vi "magnetoresistance with smu.vi"() -> ()   [LabVIEW 2017]
doc: "Use this template to build a simple state machine design pattern. Each state executes code and determines which state to transition to."
uses:
  magnetoresistance/controls/State.ctl
  <vilib>/DAQmx/create/channels.llb/DAQmx Create Channel (AI-Voltage-Basic).vi
  <vilib>/DAQmx/configure/trigger.llb/DAQmx Start Trigger (None).vi
  <vilib>/Utility/error.llb/DialogType.ctl
  <vilib>/DAQmx/write.llb/DAQmx Write (Analog DBL 1Chan 1Samp).vi
  magnetoresistance/controls/Instruments.ctl
  magnetoresistance/controls/State_of_loop.ctl
  magnetoresistance/controls/Data.ctl
  <vilib>/DAQmx/configure/timing.llb/DAQmx Timing (Sample Clock).vi
  <vilib>/DAQmx/create/channels.llb/DAQmx Create Channel (AO-Voltage-Basic).vi
panel:
  out "Type of magnet":bool
  in  "Number of loops":i32=1 caption="Stop H Field (Oe)" min=0
  in  "Time to wait, ms":i32=100 caption="Stop H Field (Oe)" min=0
  in  "Clear button":bool
  in  "Data Type":T1(ring)=enum."Resistance, Ohm"
  out "Ush.Min":dbl=-5.0
  out "Ush.Max":dbl=5.0
  out "U.Min":dbl=-5.0
  out "U.Max":dbl=5.0
  in  "Load resistance, Ohm":dbl=24000.0 min=0.0
  in  "Switch port":refnum<visa-resource-name>="COM6"
  in  "AKIP":refnum<visa-resource-name>="AKIP"
  in  "Resolution, Oe/point":dbl=100.0 caption="Stop H Field (Oe)" min=0.0 format="%#_6f"
  out "DC power electromagnet":cluster{"Voltage":dbl, "Current":dbl}={"Voltage"=0.00544, "Current"=0.05} {"Voltage" format="%.2f"; "Current" format="%.2f"}
  out "Error Out":errorcluster={"status"=FALSE, "code"=1073676293, "source"="VISA Read in AKIP_read.vi->AKIP_error_check.vi->AKIP_reset_errors.vi->magnetoresistance.vi"}
  in  "Error In (no error)":errorcluster
  in  "Voltage Output, V":dbl=2.5 min=0.0 max=5.0
  in  "H Field Max, Oe":dbl=2000.0 caption="Stop H Field (Oe)" min=0.0 max=6000.0 format="%#_6f"
  in  "H Field Min, Oe":dbl=-2000.0 min=-6000.0 max=0.0 format="%#_6f"
  out "Status":string="Shutting down..."
  in  "Exit Button":bool
  in  "Save Button":bool
  out "Cursor":cluster{"x":dbl, "y":dbl} {"x" format="%.2f"; "y" format="%.5f"}
  out "SpectrumGraph":cluster{"Old Field":dbl[], "Old Signal":dbl[]}[](graph)
  in  "Start Button":bool
  in  "Stop Button":bool
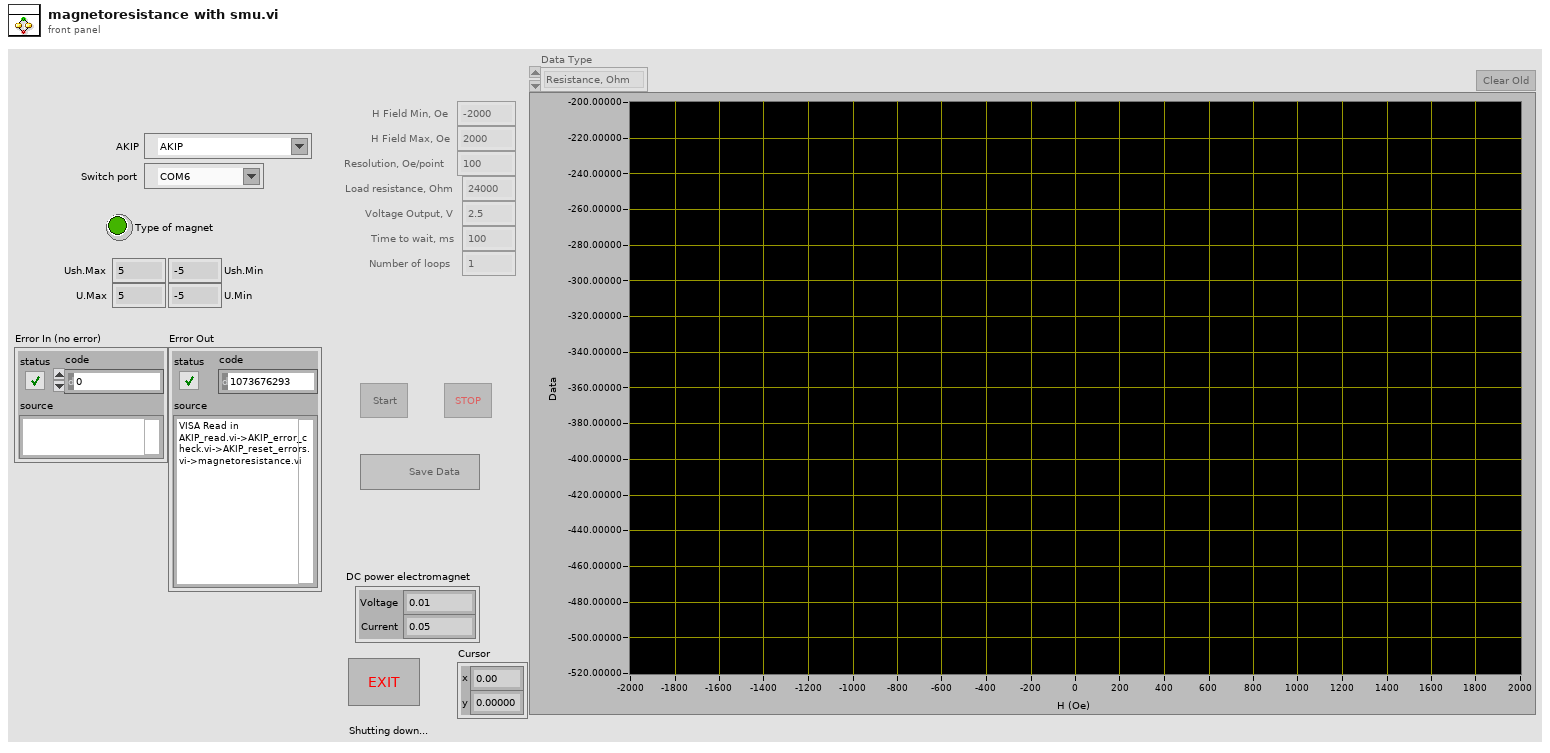
[diagram p1: front panel]
types:
  T1 = enum16{"Voltage Ush, V", "Voltage U, V", "Sum Voltage, V", "Current, mA", "Resistance, Ohm"}
  T2 = typedef "Data.ctl" = cluster{"Field":dbl[], "Voltage Ush":dbl[], "Voltage U":dbl[], "Sum Voltage":dbl[], "Current":dbl[], "Resistance":dbl[], "Old Field":dbl[], "Old Voltage Ush":dbl[], "Old Voltage U":dbl[], "Old Sum Voltage":dbl[], "Old Current":dbl[], "Old Resistance":dbl[]}
  T3 = typedef "State_of_loop.ctl" = enum16{"from zero to max", "from max to zero", "from zero to min", "from min to zero"}
  T4 = typedef "Instruments.ctl" = cluster{"DAQ AO task":refnum<k21>, "DAQ AI task":refnum<k21>, "DAQ channel Voltage Output":tag, "DAQ channel Voltage U":tag, "DAQ channel Voltage Ush":tag, "AKIP":refnum<visa-resource-name>, "Switch port":refnum<visa-resource-name>}
  T5 = typedef "State.ctl" = enum16{"Init", "Idle", "Starting meas", "Running", "Stopping meas", "Shutdown"}
  T6 = cluster{"Old Field":dbl[], "Old Resistance":dbl[]}[]
  T7 = cluster{"Voltage Ush":dbl, "Voltage U":dbl, "Sum Voltage":dbl, "Current":dbl, "Resistance":dbl}
  T8 = typedef "DialogType.ctl" = u16
  T9 = typedef "LVPoint32TypeDef.ctl" = cluster{"Horizontal":i32, "Vertical":i32}
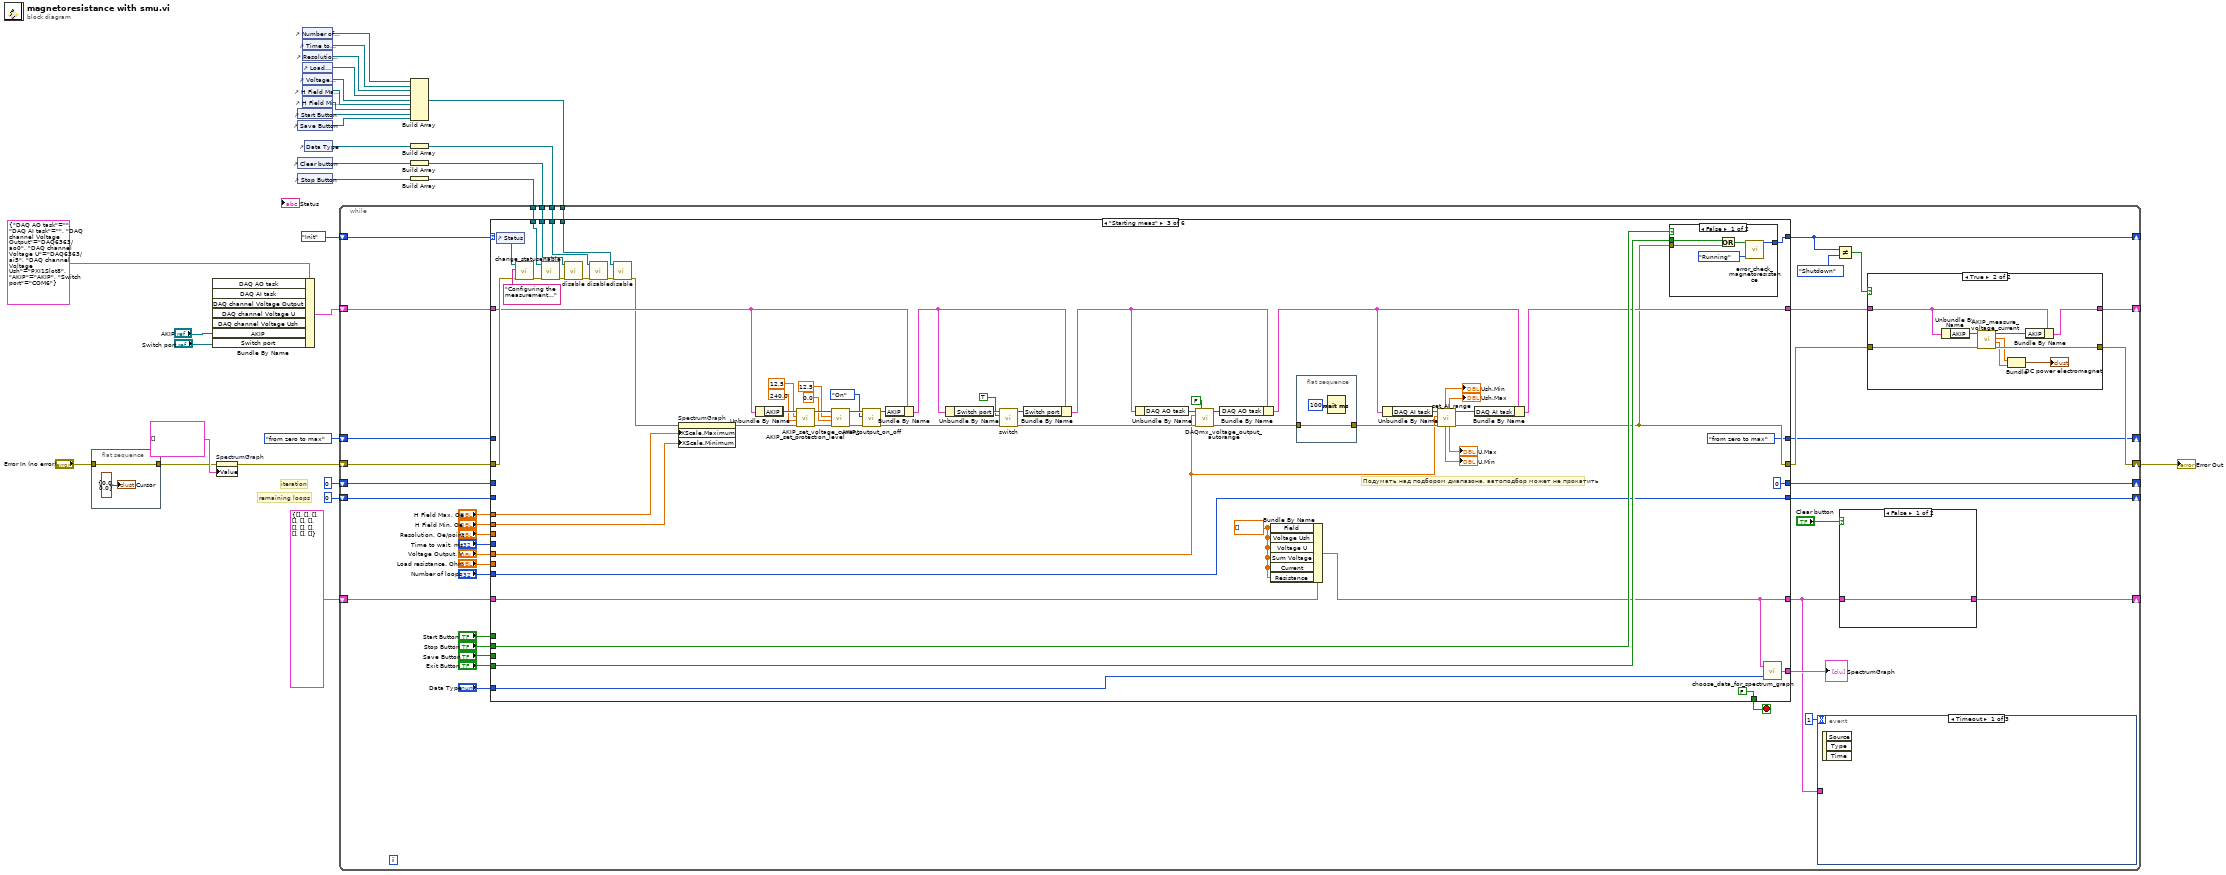
[diagram p0: block diagram]
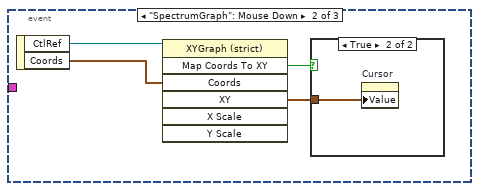
[diagram p3: hidden frame]
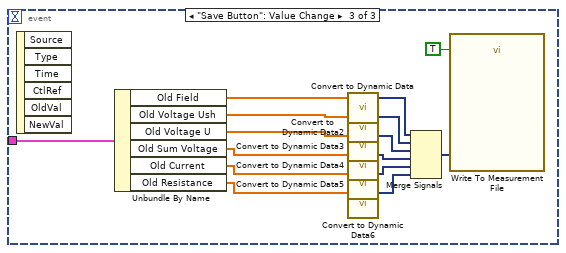
[diagram p5: hidden frame]
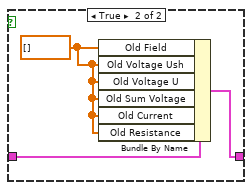
[diagram p6: hidden frame]
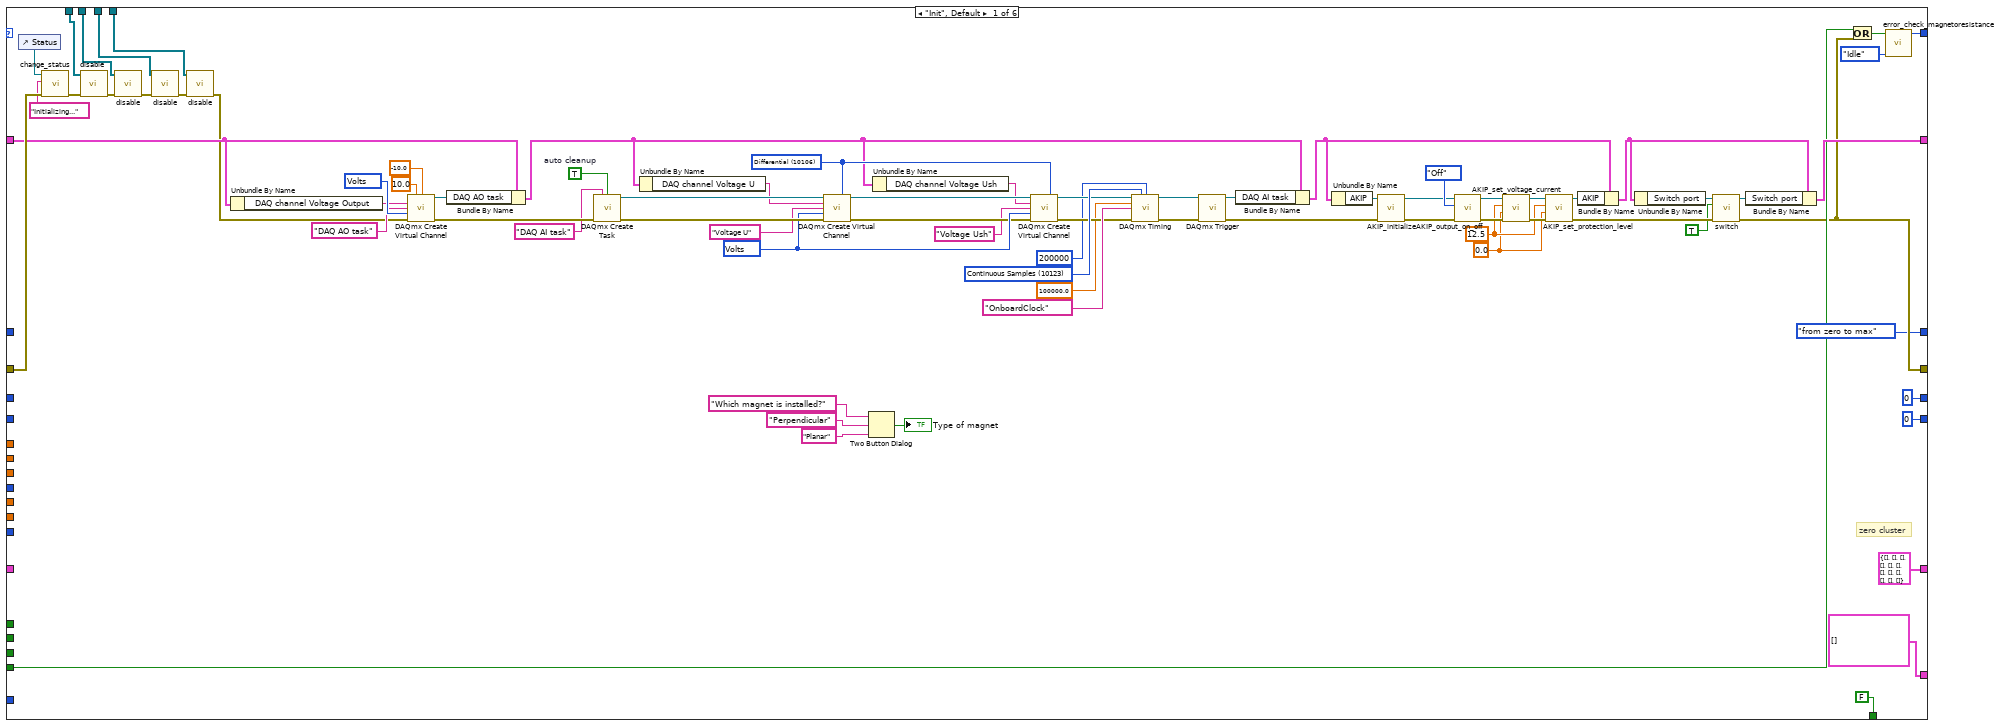
[diagram p7: hidden frame]
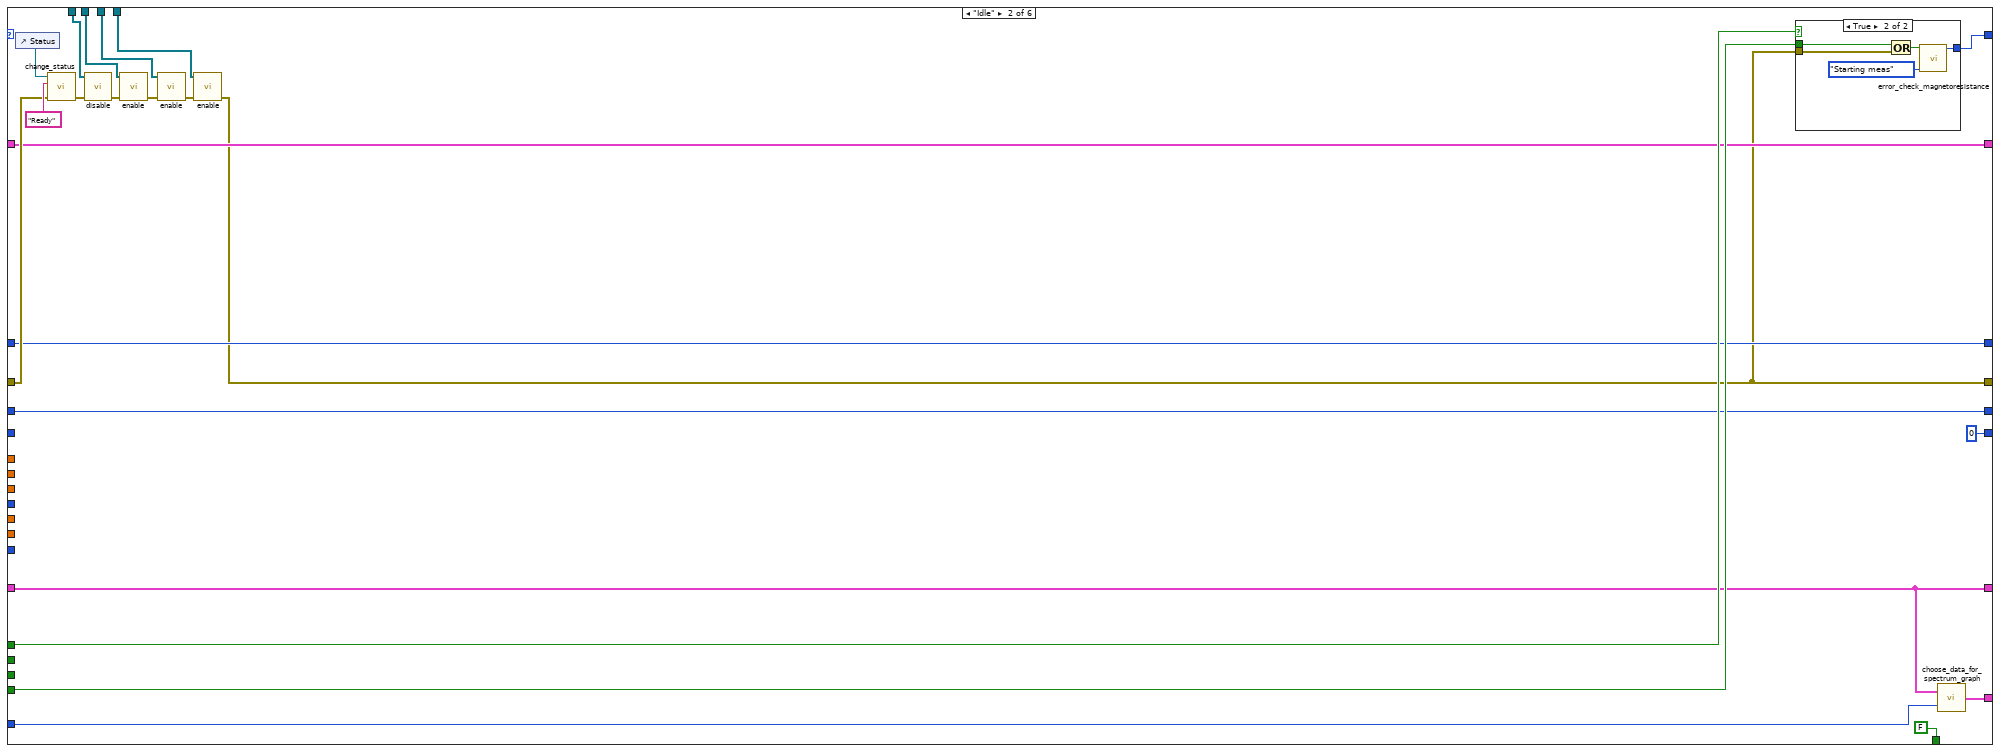
[diagram p8: hidden frame]
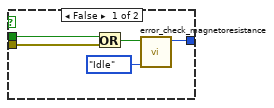
[diagram p9: hidden frame]
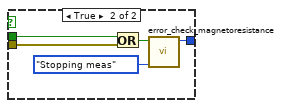
[diagram p10: hidden frame]
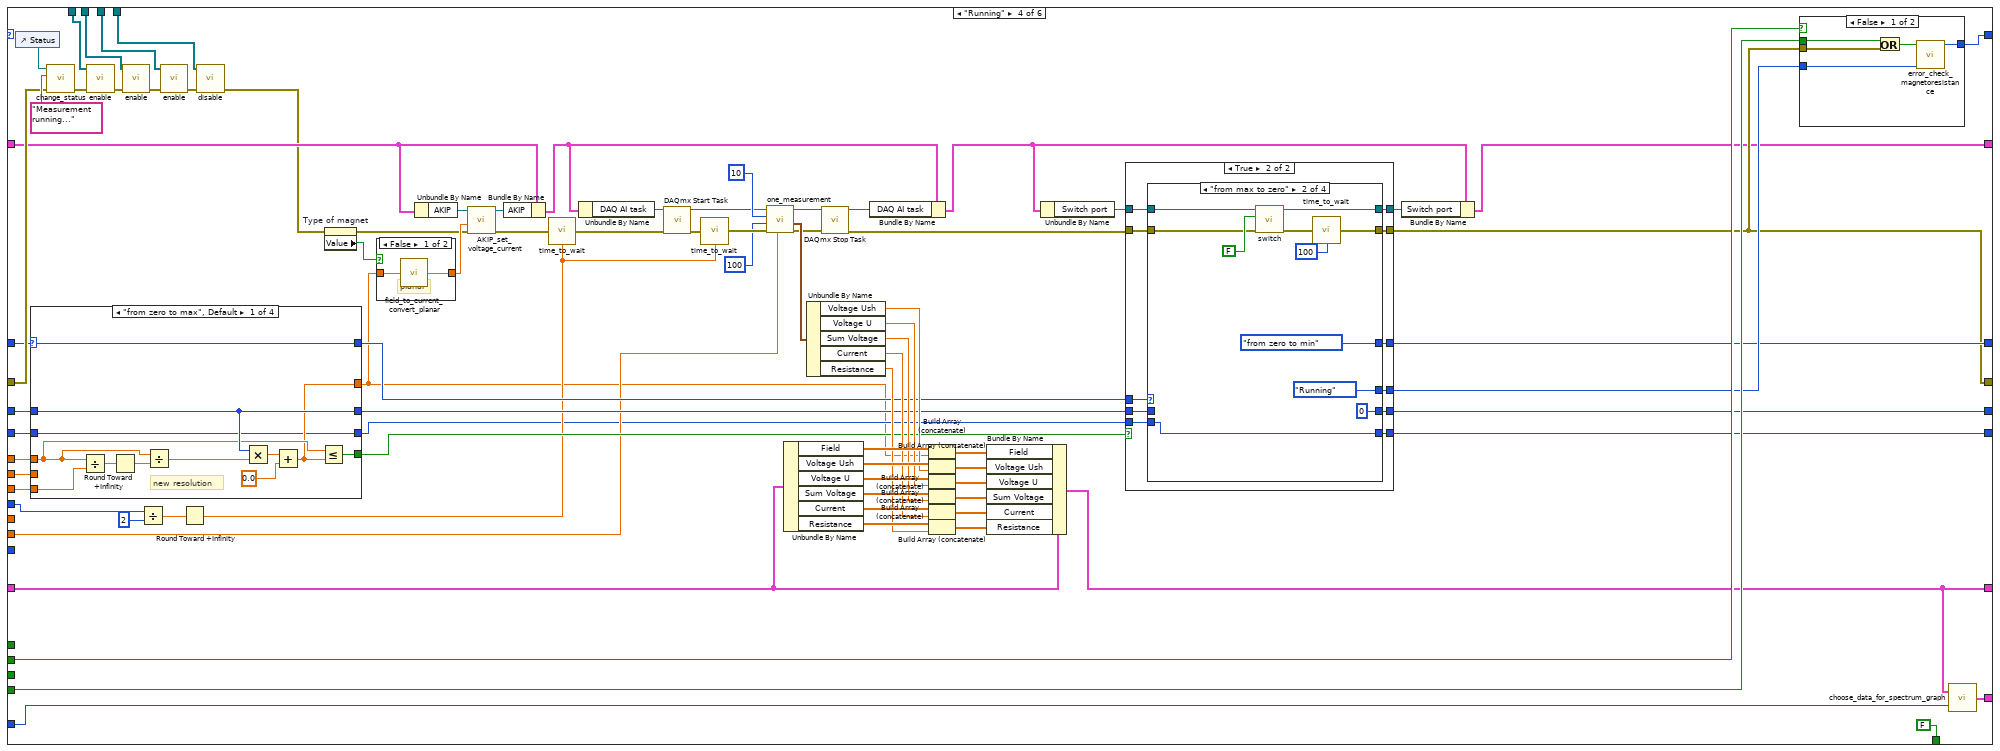
[diagram p11: hidden frame]
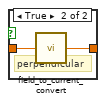
[diagram p12: hidden frame]
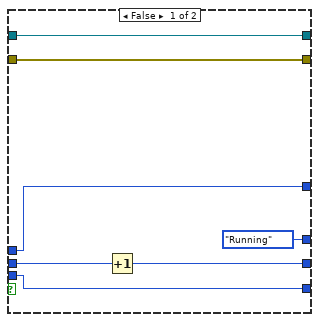
[diagram p13: hidden frame]
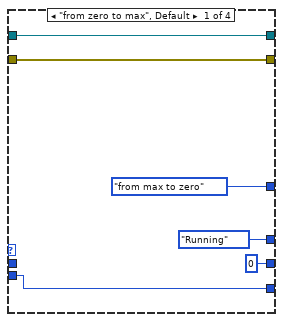
[diagram p14: hidden frame]
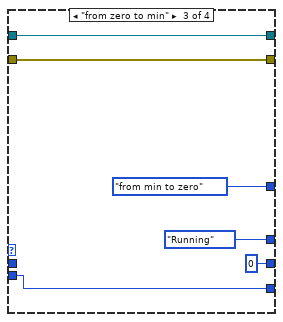
[diagram p15: hidden frame]
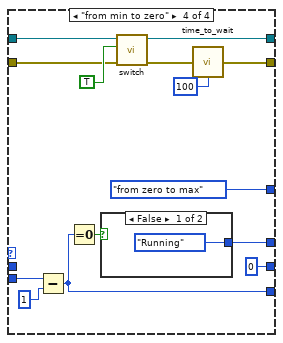
[diagram p16: hidden frame]
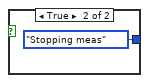
[diagram p17: hidden frame]
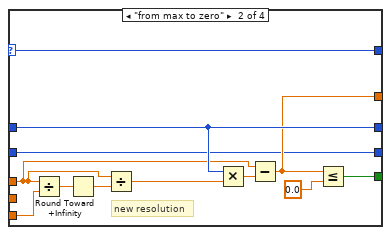
[diagram p18: hidden frame]
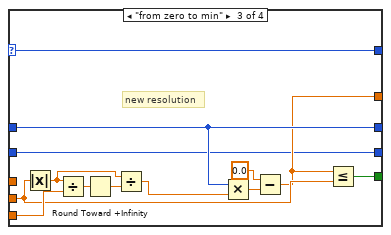
[diagram p19: hidden frame]
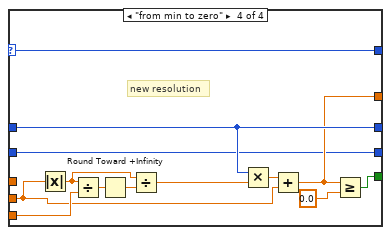
[diagram p20: hidden frame]
diagram:
  # "iteration"
  # "remaining loops"
  n1 = flat-sequence {
    tunnel: "Error In (no error)" -> [w32]
    tunnel: [w32] -> w19
    frame #0 {
      "Cursor" <- cluster{"x":dbl, "y":dbl} {"x"=0.0, "y"=0.0} ("Cursor")
    }
  }
  n2 = Bundle By Name(cluster=T4 {"DAQ AO task"="", "DAQ AI task"="", "DAQ channel Voltage Output"="DAQ6363/ao0", "DAQ channel Voltage U"="DAQ6363/ai5", "DAQ channel Voltage Ush"="PXI1Slot8", "AKIP"="AKIP", "Switch port"="COM6"} ("Cluster"), "AKIP"="AKIP", "Switch port"="Switch port") -> (w16:T4)  [unwired: 5 in]
  n3 = property on="SpectrumGraph" class="XYGraph (strict)"(error in=w19, "Value"=cluster{"Old Field":dbl[], "Old Signal":dbl[]}[] [] ("SpectrumGraph")) -> (error out=w23:errorcluster)  [unwired: 1 in, 1 out]
  n4 = control-ref of="Start Button"() -> (w28:refnum<vi>)
  n5 = control-ref of="Save Button"() -> (w27:refnum<vi>)
  n6 = control-ref of="Clear button"() -> (w10:refnum<vi>)
  n7 = control-ref of="Stop Button"() -> (w26:refnum<vi>)
  n8 = control-ref of="Number of loops"() -> (w1:refnum<vi>)
  n9 = control-ref of="Time to wait, ms"() -> (w3:refnum<vi>)
  n10 = control-ref of="Resolution, Oe/point"() -> (w4:refnum<vi>)
  n11 = control-ref of="Load resistance, Ohm"() -> (w5:refnum<vi>)
  n12 = control-ref of="Voltage Output, V"() -> (w6:refnum<vi>)
  n13 = control-ref of="H Field Max, Oe"() -> (w30:refnum<vi>)
  n14 = control-ref of="H Field Min, Oe"() -> (w29:refnum<vi>)
  n15 = control-ref of="Data Type"() -> (w9:refnum<vi>)
  n16 = Build Array(w1, w3, w4, w5, w6, w30, w29, w28, w27) -> (w24:refnum<vi>[])
  n17 = Build Array(w9) -> (w8:refnum<vi>[])
  n18 = Build Array(w10) -> (w7:refnum<vi>[])
  n19 = Build Array(w26) -> (w25:refnum<vi>[])
  n20 = while {
    tunnel: w25 -> [w71]
    tunnel: w24 -> [w70]
    shift-right: [w39] -> _
    shift-left: State."Init" ("States") -> [w64]
    shift-right: [w58] -> w15
    shift-left: w23 -> [w69]
    shift-right: [w60] -> _
    shift-left: w16 -> [w62]
    shift-right: [w51] -> _
    shift-left: State_of_loop."from zero to max" -> [w52]
    shift-right: [w49] -> _
    shift-left: 0 -> [w50]
    shift-right: [w44] -> _
    shift-left: T2 {"Field"=[], "Voltage Ush"=[], "Voltage U"=[], "Sum Voltage"=[], "Current"=[], "Resistance"=[], "Old Field"=[], "Old Voltage Ush"=[], "Old Voltage U"=[], "Old Sum Voltage"=[], "Old Current"=[], "Old Resistance"=[]} ("SpectrumGraph") -> [w48]
    tunnel: w7 -> [w41]
    tunnel: w8 -> [w40]
    shift-right: [w33] -> _
    shift-left: 0 -> [w34]
    stop <- w63 stop-if-true
    n21 = case shown="\"Starting meas\"" w64 {
      tunnel: w71 -> [w117 w187 w226 w309 w502 w552]
      tunnel: w70 -> [w114 w184 w223 w306 w499 w549]
      tunnel: w69 -> [w181 w204 w275 w368 w545 w599]
      tunnel: "Start Button" -> [_ w202 _ _ _ _]
      tunnel: "Stop Button" -> [_ _ w250 w366 _ _]
      tunnel: "Save Button" -> [_ _ _ _ _ _]
      tunnel: "Exit Button" -> [w124 w201 w249 w365 w518 _]
      tunnel: [w175 w200 w251 w367 w519 State."Shutdown" ("States out")] -> w39
      tunnel: [FALSE FALSE FALSE FALSE FALSE TRUE] -> w63
      tunnel: w62 -> [w167 w198 w240 w356 w493 w582]
      tunnel: [w125 w198 w247 w321 w497 w574] -> w61
      tunnel: [w123 w188 w246 w325 w496 w581] -> w59
      tunnel: "Load resistance, Ohm" -> [_ _ _ w297 _ _]
      tunnel: "H Field Max, Oe" -> [_ _ w220 w361 _ _]
      tunnel: "H Field Min, Oe" -> [_ _ w219 w360 _ _]
      tunnel: "Voltage Output, V" -> [_ _ w217 _ _ _]
      tunnel: "Resolution, Oe/point" -> [_ _ _ w359 _ _]
      tunnel: w52 -> [_ w197 _ w364 _ _]
      tunnel: [State_of_loop."from zero to max" w197 State_of_loop."from zero to max" w326 State_of_loop."from zero to max" State_of_loop."from zero to max"] -> w51
      tunnel: w50 -> [_ w193 _ w363 _ _]
      tunnel: [0 w193 0 w330 0 0] -> w49
      tunnel: w48 -> [_ w194 w244 w338 w509 _]
      tunnel: [T2 {"Field"=[], "Voltage Ush"=[], "Voltage U"=[], "Sum Voltage"=[], "Current"=[], "Resistance"=[], "Old Field"=[], "Old Voltage Ush"=[], "Old Voltage U"=[], "Old Sum Voltage"=[], "Old Current"=[], "Old Resistance"=[]} ("SpectrumGraph") w194 w242 w318 w508 T2 {"Field"=[], "Voltage Ush"=[], "Voltage U"=[], "Sum Voltage"=[], "Current"=[], "Resistance"=[], "Old Field"=[], "Old Voltage Ush"=[], "Old Voltage U"=[], "Old Sum Voltage"=[], "Old Current"=[], "Old Resistance"=[]} ("SpectrumGraph")] -> w43
      tunnel: [cluster{"Old Field":dbl[], "Old Signal":dbl[]}[] [] w196 w243 w320 w542 T6 [] ("Data for SpectrumGraph")] -> w47
      tunnel: "Data Type" -> [_ w195 w241 w319 w541 _]
      tunnel: w41 -> [w116 w186 w225 w308 w501 w551]
      tunnel: w40 -> [w115 w185 w224 w307 w500 w550]
      tunnel: "Time to wait, ms" -> [_ _ _ w301 _ _]
      tunnel: "Number of loops" -> [_ _ w216 _ _ _]
      tunnel: w34 -> [_ _ _ w296 _ _]
      tunnel: [0 ("Number of loops") 0 ("Number of loops") w216 w294 0 ("Number of loops") 0 ("Number of loops")] -> w33
      frame "Init", Default {
        w132 = 0.0 ("Current")
        w133 = 12.5 ("Voltage")
        w164 = TRUE  # auto cleanup
        w166 = 10123 items=["Finite Samples"=10178, "Continuous Samples"=10123, "Hardware Timed Single Point"=12522] ("sample mode")
        w157 = 10106 items=["Default"=-1, "RSE"=10083, "NRSE"=10078, "Differential"=10106, "Pseudodifferential"=12529] ("input terminal configuration")
        w156 = 10348 items=["Volts"=10348, "From Custom Scale"=10065] ("units")
        w170 = 10348 items=["Volts"=10348, "From Custom Scale"=10065] ("units")
        # "zero cluster"
        n22 = control-ref of="Status"() -> (w182:refnum<vi>)
        n23 = call "change_status.vi"("error in (no error)"=w181, "String"="Initializing...", "String in"=w182) -> ("error out"=w180:errorcluster)  [unwired: 8 in]
        n24 = call "disable.vi"("error in (no error)"=w180, "Array"=w117) -> ("error out"=w179:errorcluster)  [unwired: 9 in]
        n25 = call "disable.vi"("error in (no error)"=w179, "Array"=w116) -> ("error out"=w119:errorcluster)  [unwired: 9 in]
        n26 = call "disable.vi"("error in (no error)"=w119, "Array"=w115) -> ("error out"=w120:errorcluster)  [unwired: 9 in]
        n27 = call "disable.vi"("error in (no error)"=w120, "Array"=w114) -> ("error out"=w118:errorcluster)  [unwired: 9 in]
        n28 = Unbundle By Name(w167) -> ("DAQ channel Voltage Output"=w169:tag)
        n29 = call-poly <vilib>:"DAQmx Create Virtual Channel.vi"("maximum value"=10.0, "minimum value"=-10.0, "physical channels"=w169, "name to assign"="DAQ AO task", "units"=w170, "error in"=w118) -> ("task out"=w168:refnum<k21>, "error out"=w153:errorcluster)  [unwired: 8 in]
        n30 = Bundle By Name(cluster=w167, "DAQ AO task"=w168) -> (w143:T4)
        n31 = call <vilib>:"DAQmx Create Task.vi"("new task name"="DAQ AI task", "auto cleanup"=w164, "error in"=w153) -> ("task out"=w163:refnum<k21>, "error out"=w162:errorcluster)  [unwired: 11 in]
        n32 = Unbundle By Name(w143) -> ("DAQ channel Voltage U"=w149:tag)
        n33 = call-poly <vilib>:"DAQmx Create Virtual Channel.vi"("task in"=w163, "input terminal configuration"=w157, "physical channels"=w149, "name to assign"="Voltage U", "units"=w156, "error in"=w162) -> ("task out"=w155:refnum<k21>, "error out"=w154:errorcluster)  [unwired: 8 in]
        n34 = Two Button Dialog(message="Which magnet is installed?", 1:"Planar" ("F button name (\"Cancel\")"), 2:"Perpendicular" ("T button name (\"OK\")")) -> (T button?=→"Type of magnet":bool)
        n35 = Unbundle By Name(w143) -> ("DAQ channel Voltage Ush"=w148:tag)
        n36 = call-poly <vilib>:"DAQmx Create Virtual Channel.vi"("task in"=w155, "input terminal configuration"=w157, "physical channels"=w148, "name to assign"="Voltage Ush", "units"=w156, "error in"=w154) -> ("task out"=w161:refnum<k21>, "error out"=w160:errorcluster)  [unwired: 8 in]
        n37 = call-poly <vilib>:"DAQmx Timing.vi"("task/channels in"=w161, "sample mode"=w166, "samples per channel"=200000, "rate"=100000.0, "source"=tag "OnboardClock", "error in"=w160) -> ("task out"=w159:refnum<k21>, "error out"=w158:errorcluster)  [unwired: 8 in]
        n38 = call-poly <vilib>:"DAQmx Trigger.vi"("task/channels in"=w159, "error in"=w158) -> ("task out"=w144:refnum<k21>, "error out"=w141:errorcluster)  [unwired: 12 in]
        n39 = Bundle By Name(cluster=w143, "DAQ AI task"=w144) -> (w140:T4)
        n40 = Unbundle By Name(w140) -> ("AKIP"=w142:refnum<visa-resource-name>)
        n41 = call "AKIP_initialize.vi"("error in (no error)"=w141, "VISA Refnum in"=w142) -> ("error out"=w111:errorcluster, "VISA Refnum out"=w112:refnum<visa-resource-name>)  [unwired: 8 in]
        n42 = call "AKIP_output_on_off.vi"("error in (no error)"=w111, "Enum"=enum16{"On", "Off"}."Off", "VISA Refnum in"=w112) -> ("error out"=w136:errorcluster, "VISA Refnum out"=w137:refnum<visa-resource-name>)  [unwired: 7 in]
        n43 = call "AKIP_set_voltage_current.vi"("error in (no error)"=w136, "Current"=w132, "Voltage"=w133, "VISA resource name (in)"=w137) -> ("error out"=w135:errorcluster, "VISA resource name (out)"=w134:refnum<visa-resource-name>)  [unwired: 6 in]
        n44 = call "AKIP_set_protection_level.vi"("error in (no error)"=w135, "Current Protection Level"=w132, "Voltage Protection Level"=w133, "VISA resource name (in)"=w134) -> ("error out"=w130:errorcluster, "VISA resource name (out)"=w131:refnum<visa-resource-name>)  [unwired: 6 in]
        n45 = Bundle By Name(cluster=w140, "AKIP"=w131) -> (w126:T4)
        n46 = Unbundle By Name(w126) -> ("Switch port"=w129:refnum<visa-resource-name>)
        n47 = call "switch.vi"("error in (no error)"=w130, "Positive?"=TRUE, "Switch port (in)"=w129) -> ("error out"=w123:errorcluster, "Switch port (out)"=w127:refnum<visa-resource-name>)  [unwired: 7 in]
        n48 = Bundle By Name(cluster=w126, "Switch port"=w127) -> (w125:T4)
        n49 = Or(x=w124, y=w123) -> (x .or. y?=w176:bool)
        n50 = call "error_check_magnetoresistance.vi"("States in"=State."Idle" ("States"), "Boolean"=w176) -> ("States out"=w175:T5)  [unwired: 9 in]
      }
      frame "Idle" {
        n51 = control-ref of="Status"() -> (w203:refnum<vi>)
        n52 = call "change_status.vi"("error in (no error)"=w204, "String"="Ready", "String in"=w203) -> ("error out"=w189:errorcluster)  [unwired: 8 in]
        n53 = call "disable.vi"("error in (no error)"=w189, "Array"=w187) -> ("error out"=w192:errorcluster)  [unwired: 9 in]
        n54 = call "enable.vi"("error in (no error)"=w192, "Array"=w186) -> ("error out"=w190:errorcluster)  [unwired: 9 in]
        n55 = call "enable.vi"("error in (no error)"=w190, "Array"=w185) -> ("error out"=w191:errorcluster)  [unwired: 9 in]
        n56 = call "enable.vi"("error in (no error)"=w191, "Array"=w184) -> ("error out"=w188:errorcluster)  [unwired: 9 in]
        n57 = case shown="True" w202 {
          tunnel: w201 -> [w207 w213]
          tunnel: [w208 w212] -> w200
          tunnel: w188 -> [w206 w211]
          frame False {
            n58 = Or(x=w207, y=w206) -> (x .or. y?=w210:bool)
            n59 = call "error_check_magnetoresistance.vi"("States in"=State."Idle" ("States"), "Boolean"=w210) -> ("States out"=w208:T5)  [unwired: 9 in]
          }
          frame True {
            n60 = Or(x=w213, y=w211) -> (x .or. y?=w215:bool)
            n61 = call "error_check_magnetoresistance.vi"("States in"=State."Starting meas" ("States"), "Boolean"=w215) -> ("States out"=w212:T5)  [unwired: 9 in]
          }
        }
        n62 = call "choose_data_for_spectrum_graph.vi"("Data Type"=w195, "Data cluster"=w194) -> ("Data for SpectrumGraph"=w196:T6)
      }
      frame "Starting meas" {
        w245 = dbl[] [] ("Field")
        # "Подумать над подбором диапазона, автоподбор может не прокатить"
        n63 = control-ref of="Status"() -> (w274:refnum<vi>)
        n64 = call "change_status.vi"("error in (no error)"=w275, "String"="Configuring the measurement...", "String in"=w274) -> ("error out"=w227:errorcluster)  [unwired: 8 in]
        n65 = call "enable.vi"("error in (no error)"=w227, "Array"=w226) -> ("error out"=w230:errorcluster)  [unwired: 9 in]
        n66 = call "disable.vi"("error in (no error)"=w230, "Array"=w225) -> ("error out"=w228:errorcluster)  [unwired: 9 in]
        n67 = call "disable.vi"("error in (no error)"=w228, "Array"=w224) -> ("error out"=w229:errorcluster)  [unwired: 9 in]
        n68 = call "disable.vi"("error in (no error)"=w229, "Array"=w223) -> ("error out"=w221:errorcluster)  [unwired: 9 in]
        n69 = property on="SpectrumGraph" class="XYGraph (strict)"(error in=w221, "XScale.Maximum"=w220, "XScale.Minimum"=w219) -> (error out=w222:errorcluster)  [unwired: 1 in, 1 out]
        n70 = Unbundle By Name(w240) -> ("AKIP"=w269:refnum<visa-resource-name>)
        n71 = call "AKIP_set_protection_level.vi"("error in (no error)"=w222, "Current Protection Level"=240.0 ("Voltage Protection Level"), "Voltage Protection Level"=12.5 ("Current Protection Level"), "VISA resource name (in)"=w269) -> ("error out"=w267:errorcluster, "VISA resource name (out)"=w268:refnum<visa-resource-name>)  [unwired: 6 in]
        n72 = call "AKIP_set_voltage_current.vi"("error in (no error)"=w267, "Current"=0.0, "Voltage"=12.5, "VISA resource name (in)"=w268) -> ("error out"=w260:errorcluster, "VISA resource name (out)"=w261:refnum<visa-resource-name>)  [unwired: 6 in]
        n73 = call "AKIP_output_on_off.vi"("error in (no error)"=w260, "Enum"=enum16{"On", "Off"}."On", "VISA Refnum in"=w261) -> ("error out"=w239:errorcluster, "VISA Refnum out"=w259:refnum<visa-resource-name>)  [unwired: 7 in]
        n74 = Bundle By Name(cluster=w240, "AKIP"=w259) -> (w238:T4)
        n75 = Unbundle By Name(w238) -> ("Switch port"=w264:refnum<visa-resource-name>)
        n76 = call "switch.vi"("error in (no error)"=w239, "Positive?"=TRUE, "Switch port (in)"=w264) -> ("error out"=w218:errorcluster, "Switch port (out)"=w263:refnum<visa-resource-name>)  [unwired: 7 in]
        n77 = Bundle By Name(cluster=w238, "Switch port"=w263) -> (w237:T4)
        n78 = Unbundle By Name(w237) -> ("DAQ AO task"=w271:refnum<k21>)
        n79 = call "DAQmx_voltage_output_autorange.vi"("DAQ task Voltage Output in"=w271, "Bipolar"=FALSE, "Voltage Output, V"=w217, "error in (no error)"=w218) -> ("DAQ task Voltage Output out"=w270:refnum<k21>, "error out"=w234:errorcluster)  [unwired: 8 in, 2 out]
        n80 = Bundle By Name(cluster=w237, "DAQ AO task"=w270) -> (w248:T4)
        n81 = Bundle By Name(cluster=w244, "Field"=w245, "Voltage Ush"=w245, "Voltage U"=w245, "Sum Voltage"=w245, "Current"=w245, "Resistance"=w245) -> (w242:T2)
        n82 = flat-sequence {
          tunnel: w234 -> [w278]
          tunnel: [w278] -> w233
          frame #0 {
            n83 = Wait (ms)(milliseconds to wait=u32 100) -> ()  [unwired: 1 out]
          }
        }
        n84 = Unbundle By Name(w248) -> ("DAQ AI task"=w257:refnum<k21>)
        n85 = call "set_AI_range.vi"("error in (no error)"=w233, "Ush.Max"=w217, "U.Max"=w217, "DAQ task (in)"=w257) -> ("error out"=w246:errorcluster, "DAQ task (out)"=w256:refnum<k21>, "U.Max"=→"U.Max":dbl, "Ush.Max"=→"Ush.Max":dbl, "U.Min"=→"U.Min":dbl, "Ush.Min"=→"Ush.Min":dbl)  [unwired: 2 in]
        n86 = Bundle By Name(cluster=w248, "DAQ AI task"=w256) -> (w247:T4)
        n87 = case shown="False" w250 {
          tunnel: w249 -> [w280 w286]
          tunnel: [w281 w285] -> w251
          tunnel: w246 -> [w279 w284]
          frame False {
            n88 = Or(x=w280, y=w279) -> (x .or. y?=w283:bool)
            n89 = call "error_check_magnetoresistance.vi"("States in"=State."Running" ("States"), "Boolean"=w283) -> ("States out"=w281:T5)  [unwired: 9 in]
          }
          frame True {
            n90 = Or(x=w286, y=w284) -> (x .or. y?=w288:bool)
            n91 = call "error_check_magnetoresistance.vi"("States in"=State."Stopping meas" ("States"), "Boolean"=w288) -> ("States out"=w285:T5)  [unwired: 9 in]
          }
        }
        n92 = call "choose_data_for_spectrum_graph.vi"("Data Type"=w241, "Data cluster"=w242) -> ("Data for SpectrumGraph"=w243:T6)
      }
      frame "Running" {
        n93 = control-ref of="Status"() -> (w369:refnum<vi>)
        n94 = case shown="\"from zero to max\", Default" w364 {
          selector: w364 -> [w433 w445 w457 w470]
          tunnel: w363 -> [w443 w451 w462 w476]
          tunnel: [w443 w451 w462 w476] -> w331
          tunnel: w361 -> [w435 w449 _ _]
          tunnel: w360 -> [_ _ w460 w474]
          tunnel: w359 -> [w438 w452 w464 w477]
          tunnel: [w434 w446 w458 w471] -> w292
          tunnel: [w436 w447 w459 w472] -> w328
          tunnel: [w433 w445 w457 w470] -> w327
          tunnel: w296 -> [w432 w444 w456 w469]
          tunnel: [w432 w444 w456 w469] -> w295
          frame "from zero to max", Default {
            # "new resolution"
            n95 = Divide(x=w435, y=w438) -> (x/y=w439:dbl)
            n96 = Round Toward +Infinity(x=w439) -> (ceil(x): smallest int >= x=w440:dbl)
            n97 = Divide(x=w435, y=w440) -> (x/y=w437:dbl)
            n98 = Multiply(x=w443, y=w437) -> (x*y=w442:dbl)
            n99 = Add(x=w442, y=0.0) -> (x+y=w434:dbl)
            n100 = Less Or Equal?(x=w435, y=w434) -> (x <= y?=w436:bool)
          }
          frame "from max to zero" {
            # "new resolution"
            n101 = Divide(x=w449, y=w452) -> (x/y=w454:dbl)
            n102 = Round Toward +Infinity(x=w454) -> (ceil(x): smallest int >= x=w453:dbl)
            n103 = Divide(x=w449, y=w453) -> (x/y=w455:dbl)
            n104 = Multiply(x=w451, y=w455) -> (x*y=w450:dbl)
            n105 = Subtract(x=w449, y=w450) -> (x-y=w446:dbl)
            n106 = Less Or Equal?(x=w446, y=0.0) -> (x <= y?=w447:bool)
          }
          frame "from zero to min" {
            # "new resolution"
            n107 = Absolute Value(x=w460) -> (abs(x)=w463:dbl)
            n108 = Divide(x=w463, y=w464) -> (x/y=w467:dbl)
            n109 = Round Toward +Infinity(x=w467) -> (ceil(x): smallest int >= x=w466:dbl)
            n110 = Divide(x=w463, y=w466) -> (x/y=w468:dbl)
            n111 = Multiply(x=w462, y=w468) -> (x*y=w465:dbl)
            n112 = Subtract(x=0.0, y=w465) -> (x-y=w458:dbl)
            n113 = Less Or Equal?(x=w458, y=w460) -> (x <= y?=w459:bool)
          }
          frame "from min to zero" {
            # "new resolution"
            n114 = Absolute Value(x=w474) -> (abs(x)=w478:dbl)
            n115 = Divide(x=w478, y=w477) -> (x/y=w480:dbl)
            n116 = Round Toward +Infinity(x=w480) -> (ceil(x): smallest int >= x=w479:dbl)
            n117 = Divide(x=w478, y=w479) -> (x/y=w481:dbl)
            n118 = Multiply(x=w476, y=w481) -> (x*y=w475:dbl)
            n119 = Add(x=w475, y=w474) -> (x+y=w471:dbl)
            n120 = Greater Or Equal?(x=w471, y=0.0) -> (x >= y?=w472:bool)
          }
        }
        n121 = call "change_status.vi"("error in (no error)"=w368, "String"="Measurement running...", "String in"=w369) -> ("error out"=w310:errorcluster)  [unwired: 8 in]
        n122 = call "enable.vi"("error in (no error)"=w310, "Array"=w309) -> ("error out"=w313:errorcluster)  [unwired: 9 in]
        n123 = call "enable.vi"("error in (no error)"=w313, "Array"=w308) -> ("error out"=w311:errorcluster)  [unwired: 9 in]
        n124 = Divide(x=w301, y=2) -> (x/y=w299:dbl)
        n125 = call "enable.vi"("error in (no error)"=w311, "Array"=w307) -> ("error out"=w312:errorcluster)  [unwired: 9 in]
        n126 = Round Toward +Infinity(x=w299) -> (ceil(x): smallest int >= x=w298:dbl)
        n127 = call "disable.vi"("error in (no error)"=w312, "Array"=w306) -> ("error out"=w291:errorcluster)  [unwired: 9 in]
        n128 = property on="Type of magnet" class="Bool (strict)"(error in=w291) -> (error out=w290:errorcluster, "Value"=w289:bool)  [unwired: 1 in, 1 out]
        n129 = case shown="False" w289 {
          tunnel: w292 -> [w372 w374]
          tunnel: [w371 w373] -> w293
          frame False {
            # "planar"
            n130 = call "field_to_current_convert_planar.vi"("Field, Oe"=w372) -> ("Current, A"=w371:dbl)
          }
          frame True {
            # "perpendicular"
            n131 = call "field_to_current_convert.vi"("Field, Oe"=w374) -> ("Current, A"=w373:dbl)
          }
        }
        n132 = Unbundle By Name(w356) -> ("AKIP"=w358:refnum<visa-resource-name>)
        n133 = call "AKIP_set_voltage_current.vi"("error in (no error)"=w290, "Current"=w293, "VISA resource name (in)"=w358) -> ("error out"=w303:errorcluster, "VISA resource name (out)"=w357:refnum<visa-resource-name>)  [unwired: 7 in]
        n134 = Bundle By Name(cluster=w356, "AKIP"=w357) -> (w353:T4)
        n135 = call "time_to_wait.vi"("error in (no error)"=w303, "milliseconds to wait"=w298) -> ("error out"=w302:errorcluster)
        n136 = Unbundle By Name(w353) -> ("DAQ AI task"=w355:refnum<k21>)
        n137 = call <vilib>:"DAQmx Start Task.vi"("task/channels in"=w355, "error in"=w302) -> ("task out"=w305:refnum<k21>, "error out"=w304:errorcluster)  [unwired: 12 in]
        n138 = call "time_to_wait.vi"("error in (no error)"=w304, "milliseconds to wait"=w298) -> ("error out"=w354:errorcluster)
        n139 = call "one_measurement.vi"("Rsh, Ohm"=w297, "Error (in)"=w354, "Number of points"=100, "time for one scan, ms"=u32 10, "DAQ AI task (in)"=w305) -> ("Error (out)"=w315:errorcluster, "Data"=w344:T7, "DAQ AI task (out)"=w317:refnum<k21>)  [unwired: 4 in]
        n140 = Unbundle By Name(w338) -> ("Field"=w350:dbl[], "Voltage Ush"=w349:dbl[], "Voltage U"=w348:dbl[], "Sum Voltage"=w347:dbl[], "Current"=w346:dbl[], "Resistance"=w345:dbl[])
        n141 = Unbundle By Name(w344) -> ("Voltage Ush"=w343:dbl, "Voltage U"=w342:dbl, "Sum Voltage"=w341:dbl, "Current"=w340:dbl, "Resistance"=w339:dbl)
        n142 = call <vilib>:"DAQmx Stop Task.vi"("task/channels in"=w317, "error in"=w315) -> ("task out"=w316:refnum<k21>, "error out"=w314:errorcluster)  [unwired: 12 in]
        n143 = Bundle By Name(cluster=w353, "DAQ AI task"=w316) -> (w322:T4)
        n144 = Build Array (concatenate)(w350, w292) -> (w337:dbl[])
        n145 = Build Array (concatenate)(w349, w343) -> (w336:dbl[])
        n146 = Build Array (concatenate)(w348, w342) -> (w335:dbl[])
        n147 = Build Array (concatenate)(w347, w341) -> (w334:dbl[])
        n148 = Build Array (concatenate)(w346, w340) -> (w333:dbl[])
        n149 = Build Array (concatenate)(w345, w339) -> (w332:dbl[])
        n150 = Bundle By Name(cluster=w338, "Field"=w337, "Voltage Ush"=w336, "Voltage U"=w335, "Sum Voltage"=w334, "Current"=w333, "Resistance"=w332) -> (w318:T2)
        n151 = Unbundle By Name(w322) -> ("Switch port"=w324:refnum<visa-resource-name>)
        n152 = case shown="True" w328 {
          tunnel: w331 -> [w380 w390]
          tunnel: [w379 w389] -> w330
          tunnel: [State."Running" ("States") w388] -> w329
          tunnel: w327 -> [w378 w392]
          tunnel: [w378 w391] -> w326
          tunnel: w314 -> [w376 w387]
          tunnel: [w376 w386] -> w325
          tunnel: w324 -> [w377 w385]
          tunnel: [w377 w384] -> w323
          tunnel: w295 -> [w375 w383]
          tunnel: [w375 w382] -> w294
          frame False {
            n153 = Increment(x=w380) -> (x+1=w379:i32)
          }
          frame True {
            n154 = case shown="\"from max to zero\"" w392 {
              tunnel: [State_of_loop."from max to zero" State_of_loop."from zero to min" State_of_loop."from min to zero" State_of_loop."from zero to max"] -> w391
              tunnel: w390 -> [_ _ _ _]
              tunnel: [0 0 0 0] -> w389
              tunnel: [State."Running" ("States") State."Running" ("States") State."Running" ("States") w428] -> w388
              tunnel: w387 -> [w396 w405 w413 w426]
              tunnel: [w396 w400 w413 w420] -> w386
              tunnel: w385 -> [w395 w406 w412 w425]
              tunnel: [w395 w404 w412 w424] -> w384
              tunnel: w383 -> [w393 w399 w410 w419]
              tunnel: [w393 w399 w410 w416] -> w382
              frame "from zero to max", Default {
              }
              frame "from max to zero" {
                n155 = call "switch.vi"("error in (no error)"=w405, "Positive?"=FALSE, "Switch port (in)"=w406) -> ("error out"=w401:errorcluster, "Switch port (out)"=w404:refnum<visa-resource-name>)  [unwired: 7 in]
                n156 = call "time_to_wait.vi"("error in (no error)"=w401, "milliseconds to wait"=u32 100) -> ("error out"=w400:errorcluster)
              }
              frame "from zero to min" {
              }
              frame "from min to zero" {
                n157 = Subtract(x=w419, y=1) -> (x-y=w416:i32)
                n158 = Equal To 0?(x=w416) -> (x = 0?=w417:bool)
                n159 = case shown="False" w417 {
                  tunnel: [State."Running" ("States") State."Stopping meas" ("States")] -> w428
                  frame False {
                  }
                  frame True {
                  }
                }
                n160 = call "switch.vi"("error in (no error)"=w426, "Positive?"=TRUE, "Switch port (in)"=w425) -> ("error out"=w421:errorcluster, "Switch port (out)"=w424:refnum<visa-resource-name>)  [unwired: 7 in]
                n161 = call "time_to_wait.vi"("error in (no error)"=w421, "milliseconds to wait"=u32 100) -> ("error out"=w420:errorcluster)
              }
            }
          }
        }
        n162 = Bundle By Name(cluster=w322, "Switch port"=w323) -> (w321:T4)
        n163 = case shown="False" w366 {
          tunnel: w365 -> [w484 w489]
          tunnel: [w485 w488] -> w367
          tunnel: w325 -> [w483 w487]
          tunnel: w329 -> [w482 _]
          frame False {
            n164 = Or(x=w484, y=w483) -> (x .or. y?=w486:bool)
            n165 = call "error_check_magnetoresistance.vi"("States in"=w482, "Boolean"=w486) -> ("States out"=w485:T5)  [unwired: 9 in]
          }
          frame True {
            n166 = Or(x=w489, y=w487) -> (x .or. y?=w491:bool)
            n167 = call "error_check_magnetoresistance.vi"("States in"=State."Stopping meas" ("States"), "Boolean"=w491) -> ("States out"=w488:T5)  [unwired: 9 in]
          }
        }
        n168 = call "choose_data_for_spectrum_graph.vi"("Data Type"=w319, "Data cluster"=w318) -> ("Data for SpectrumGraph"=w320:T6)
      }
      frame "Stopping meas" {
        w507 = dbl[] [] ("Field")
        n169 = control-ref of="Status"() -> (w544:refnum<vi>)
        n170 = call "change_status.vi"("error in (no error)"=w545, "String"="Stopping the measurement...", "String in"=w544) -> ("error out"=w503:errorcluster)  [unwired: 8 in]
        n171 = call "disable.vi"("error in (no error)"=w503, "Array"=w502) -> ("error out"=w506:errorcluster)  [unwired: 9 in]
        n172 = call "disable.vi"("error in (no error)"=w506, "Array"=w501) -> ("error out"=w504:errorcluster)  [unwired: 9 in]
        n173 = call "disable.vi"("error in (no error)"=w504, "Array"=w500) -> ("error out"=w505:errorcluster)  [unwired: 9 in]
        n174 = call "disable.vi"("error in (no error)"=w505, "Array"=w499) -> ("error out"=w494:errorcluster)  [unwired: 9 in]
        n175 = Unbundle By Name(w493) -> ("DAQ AO task"=w524:refnum<k21>)
        n176 = call-poly <vilib>:"DAQmx Write.vi"("task/channels in"=w524, "data"=0.0 ("Voltage Output, V"), "error in"=w494) -> ("task out"=w523:refnum<k21>, "error out"=w495:errorcluster)  [unwired: 10 in, 1 out]
        n177 = Bundle By Name(cluster=w493, "DAQ AO task"=w523) -> (w492:T4)
        n178 = Unbundle By Name(w492) -> ("AKIP"=w540:refnum<visa-resource-name>)
        n179 = call "AKIP_set_voltage_current.vi"("error in (no error)"=w495, "Current"=0.0 ("Voltage Protection Level"), "Voltage"=12.5 ("Current Protection Level"), "VISA resource name (in)"=w540) -> ("error out"=w538:errorcluster, "VISA resource name (out)"=w539:refnum<visa-resource-name>)  [unwired: 6 in]
        n180 = call "AKIP_set_protection_level.vi"("error in (no error)"=w538, "Current Protection Level"=0.0 ("Current"), "Voltage Protection Level"=12.5 ("Voltage"), "VISA resource name (in)"=w539) -> ("error out"=w531:errorcluster, "VISA resource name (out)"=w532:refnum<visa-resource-name>)  [unwired: 6 in]
        n181 = call "AKIP_output_on_off.vi"("error in (no error)"=w531, "Enum"=enum16{"On", "Off"}."Off", "VISA Refnum in"=w532) -> ("error out"=w528:errorcluster, "VISA Refnum out"=w530:refnum<visa-resource-name>)  [unwired: 7 in]
        n182 = Bundle By Name(cluster=w492, "AKIP"=w530) -> (w527:T4)
        n183 = Unbundle By Name(w527) -> ("Switch port"=w535:refnum<visa-resource-name>)
        n184 = call "switch.vi"("error in (no error)"=w528, "Positive?"=TRUE, "Switch port (in)"=w535) -> ("error out"=w496:errorcluster, "Switch port (out)"=w534:refnum<visa-resource-name>)  [unwired: 7 in]
        n185 = Bundle By Name(cluster=w527, "Switch port"=w534) -> (w497:T4)
        n186 = Unbundle By Name(w509) -> ("Field"=w515:dbl[], "Voltage Ush"=w514:dbl[], "Voltage U"=w513:dbl[], "Sum Voltage"=w512:dbl[], "Current"=w511:dbl[], "Resistance"=w510:dbl[])
        n187 = Bundle By Name(cluster=w509, "Field"=w507, "Voltage Ush"=w507, "Voltage U"=w507, "Sum Voltage"=w507, "Current"=w507, "Resistance"=w507, "Old Field"=w515, "Old Voltage Ush"=w514, "Old Voltage U"=w513, "Old Sum Voltage"=w512, "Old Current"=w511, "Old Resistance"=w510) -> (w508:T2)
        n188 = Or(x=w518, y=w496) -> (x .or. y?=w521:bool)
        n189 = call "error_check_magnetoresistance.vi"("States in"=State."Idle" ("States"), "Boolean"=w521) -> ("States out"=w519:T5)  [unwired: 9 in]
        n190 = call "choose_data_for_spectrum_graph.vi"("Data Type"=w541, "Data cluster"=w508) -> ("Data for SpectrumGraph"=w542:T6)
      }
      frame "Shutdown" {
        w564 = 12.5 ("Voltage")
        w563 = 0.0 ("Current")
        w595 = T8 3 items=["no dialog", "OK message", "continue or stop message", "OK message + warnings", "continue/stop + warnings"] ("type of dialog (OK msg:1)")
        # "zero cluster"
        n191 = control-ref of="Status"() -> (w598:refnum<vi>)
        n192 = call "change_status.vi"("error in (no error)"=w599, "String"="Shutting down...", "String in"=w598) -> ("error out"=w553:errorcluster)  [unwired: 8 in]
        n193 = call "disable.vi"("error in (no error)"=w553, "Array"=w552) -> ("error out"=w556:errorcluster)  [unwired: 9 in]
        n194 = call "disable.vi"("error in (no error)"=w556, "Array"=w551) -> ("error out"=w554:errorcluster)  [unwired: 9 in]
        n195 = call "disable.vi"("error in (no error)"=w554, "Array"=w550) -> ("error out"=w555:errorcluster)  [unwired: 9 in]
        n196 = call "disable.vi"("error in (no error)"=w555, "Array"=w549) -> ("error out"=w548:errorcluster)  [unwired: 9 in]
        n197 = Unbundle By Name(w582) -> ("DAQ AI task"=w587:refnum<k21>)
        n198 = call <vilib>:"DAQmx Stop Task.vi"("task/channels in"=w587, "error in"=w548) -> ("task out"=w596:refnum<k21>, "error out"=w597:errorcluster)  [unwired: 12 in]
        n199 = call <vilib>:"DAQmx Clear Task.vi"("task in"=w596, "error in"=w597) -> ("error out"=w588:errorcluster)  [unwired: 13 in]
        n200 = Unbundle By Name(w582) -> ("DAQ AO task"=w586:refnum<k21>)
        n201 = call-poly <vilib>:"DAQmx Write.vi"("task/channels in"=w586, "auto start"=TRUE, "data"=0.0, "error in"=w588) -> ("task out"=w591:refnum<k21>, "error out"=w592:errorcluster)  [unwired: 9 in, 1 out]
        n202 = call <vilib>:"DAQmx Stop Task.vi"("task/channels in"=w591, "error in"=w592) -> ("task out"=w593:refnum<k21>, "error out"=w594:errorcluster)  [unwired: 12 in]
        n203 = call <vilib>:"DAQmx Clear Task.vi"("task in"=w593, "error in"=w594) -> ("error out"=w566:errorcluster)  [unwired: 13 in]
        n204 = Unbundle By Name(w582) -> ("AKIP"=w565:refnum<visa-resource-name>)
        n205 = call "AKIP_set_voltage_current.vi"("error in (no error)"=w566, "Current"=w563, "Voltage"=w564, "VISA resource name (in)"=w565) -> ("error out"=w568:errorcluster, "VISA resource name (out)"=w567:refnum<visa-resource-name>)  [unwired: 6 in]
        n206 = call "AKIP_set_protection_level.vi"("error in (no error)"=w568, "Current Protection Level"=w563, "Voltage Protection Level"=w564, "VISA resource name (in)"=w567) -> ("error out"=w561:errorcluster, "VISA resource name (out)"=w562:refnum<visa-resource-name>)  [unwired: 6 in]
        n207 = call "AKIP_output_on_off.vi"("error in (no error)"=w561, "Enum"=enum16{"On", "Off"}."Off", "VISA Refnum in"=w562) -> ("error out"=w559:errorcluster, "VISA Refnum out"=w560:refnum<visa-resource-name>)  [unwired: 7 in]
        n208 = call "AKIP_reset_errors.vi"("error in (no error)"=w559, "VISA Refnum in"=w560) -> ("error out"=w584:errorcluster, "VISA Refnum out"=w585:refnum<visa-resource-name>)  [unwired: 8 in]
        n209 = call "AKIP_close.vi"("error in (no error)"=w584, "VISA Refnum in"=w585) -> ("error out"=w579:errorcluster, "VISA resource name out"=w583:refnum<visa-resource-name>)  [unwired: 8 in]
        n210 = Bundle By Name(cluster=w582, "AKIP"=w583) -> (w575:T4)
        n211 = Unbundle By Name(w575) -> ("Switch port"=w578:refnum<visa-resource-name>)
        n212 = call "switch.vi"("error in (no error)"=w579, "Positive?"=TRUE, "Switch port (in)"=w578) -> ("error out"=w573:errorcluster, "Switch port (out)"=w576:refnum<visa-resource-name>)  [unwired: 7 in]
        n213 = Bundle By Name(cluster=w575, "Switch port"=w576) -> (w574:T4)
        n214 = call <vilib>:"Simple Error Handler.vi"("type of dialog (OK msg:1)"=w595, "error in (no error)"=w573) -> ("error out"=w581:errorcluster)  [unwired: 3 in, 4 out]
      }
    }
    "SpectrumGraph" <- w47
    n215 = event shown="[0] Timeout" {
      selector: _ -> [_ _ _]
      dyn-events: _ -> [_ _ _]
      timeout: 1 -> [_ _ _]
      tunnel: w43 -> [_ _ w95]
      event Timeout {
        n216 = event-data() -> ()  [unwired: 1 in, 3 out]
      }
      event "SpectrumGraph": Mouse Down {
        n217 = event-data() -> ("CtlRef"=w84:refnum<vi>, "Coords"=w83:T9)  [unwired: 1 in]
        n218 = invoke on="Invoke Node" class="XYGraph (strict)" method="Map Coords To XY"(reference=w84, "Coords"=w83) -> ("Map Coords To XY"=w85:bool, "XY"=w86:cluster{"X":dbl, "Y":dbl})  [unwired: 5 in, 5 out]
        n219 = case shown="True" w85 {
          tunnel: w86 -> [_ w87]
          frame False {
          }
          frame True {
            n220 = property on="Cursor" class="Clust (strict)"("Value"=w87) -> ()  [unwired: 2 in, 2 out]
          }
        }
      }
      event "Save Button": Value Change {
        n221 = event-data() -> ()  [unwired: 1 in, 6 out]
        n222 = Unbundle By Name(w95) -> ("Old Field"=w102:dbl[], "Old Voltage Ush"=w100:dbl[], "Old Voltage U"=w96:dbl[], "Old Sum Voltage"=w94:dbl[], "Old Current"=w93:dbl[], "Old Resistance"=w92:dbl[])
        n223 = call "Convert to Dynamic Data"("Array"=w102) -> ("Dynamic Data Type"=w101:dynamicdata)  [unwired: 3 in]
        n224 = call "Convert to Dynamic Data2"("Array"=w100) -> ("Dynamic Data Type"=w99:dynamicdata)  [unwired: 3 in]
        n225 = call "Convert to Dynamic Data3"("Array"=w96) -> ("Dynamic Data Type"=w97:dynamicdata)  [unwired: 3 in]
        n226 = call "Convert to Dynamic Data4"("Array"=w94) -> ("Dynamic Data Type"=w91:dynamicdata)  [unwired: 3 in]
        n227 = call "Convert to Dynamic Data5"("Array"=w93) -> ("Dynamic Data Type"=w90:dynamicdata)  [unwired: 3 in]
        n228 = call "Convert to Dynamic Data6"("Array"=w92) -> ("Dynamic Data Type"=w89:dynamicdata)  [unwired: 3 in]
        n229 = Merge Signals(w101, w99, w97, w91, w90, w89) -> (w98:dynamicdata)
        n230 = call "Write To Measurement File"("Signals"=w98, "Reset"=TRUE) -> ()  [unwired: 15 in, 3 out]
      }
    }
    n231 = Not Equal?(x=w39, y=State."Shutdown") -> (x != y?=w37:bool)
    n232 = case shown="False" "Clear button" {
      tunnel: w43 -> [w103 w106]
      tunnel: [w103 w105] -> w44
      frame False {
      }
      frame True {
        w104 = dbl[] [] ("Old Field")
        n233 = Bundle By Name(cluster=w106, "Old Field"=w104, "Old Voltage Ush"=w104, "Old Voltage U"=w104, "Old Sum Voltage"=w104, "Old Current"=w104, "Old Resistance"=w104) -> (w105:T2)
      }
    }
    n234 = case shown="True" w37 {
      tunnel: w61 -> [w73 w80]
      tunnel: [w73 w79] -> w60
      tunnel: w59 -> [w72 w78]
      tunnel: [w72 w77] -> w58
      frame False {
      }
      frame True {
        n235 = Unbundle By Name(w80) -> ("AKIP"=w82:refnum<visa-resource-name>)
        n236 = call "AKIP_measure_voltage_current.vi"("error in (no error)"=w78, "VISA Refnum in"=w82) -> ("error out"=w77:errorcluster, "Current"=w75:dbl, "Voltage"=w76:dbl, "VISA Refnum out"=w81:refnum<visa-resource-name>)  [unwired: 6 in]
        n237 = Bundle("Voltage"=w76, "Current"=w75) -> (→"DC power electromagnet":cluster{"Voltage":dbl, "Current":dbl})  [unwired: 1 in]
        n238 = Bundle By Name(cluster=w80, "AKIP"=w81) -> (w79:T4)
      }
    }
  }
  "Error Out" <- w15
